vi "点在矩形中（TB）.vi"(11 "point":cluster{"x":i16, "y":i16} caption="点") -> (3 "pt in rect":bool caption="矩形中的点")   [LabVIEW 2012]
uses:
  RectTB.ctl
panel:
  in  "RectTB":T1
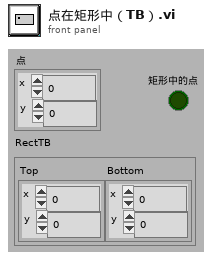
[diagram p1: front panel]
types:
  T1 = typedef "RectTB.ctl" = cluster{"Top":cluster{"x":i16, "y":i16}, "Bottom":cluster{"x":i16, "y":i16}}
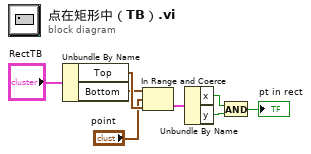
[diagram p0: block diagram]
diagram:
  n1 = Unbundle By Name("RectTB") -> ("Top"=w8:cluster{"x":i16, "y":i16}, "Bottom"=w7:cluster{"x":i16, "y":i16})
  n2 = In Range and Coerce(upper limit=w7, x="point", lower limit=w8) -> (In Range?=w5:cluster{"x":bool, "y":bool})  [unwired: 1 out]
  n3 = Unbundle By Name(w5) -> ("x"=w4:bool, "y"=w3:bool)
  n4 = And(x=w4, y=w3) -> (x .and. y?=→"pt in rect":bool)
